vi "Mem_LvDataToMemory.vi"   [LabVIEW 2019, in "Memory Data Access.lvlib"]
uses:
  Memory Data Access.lvlib
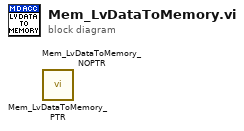
[diagram p0: block diagram]
diagram:
  n1 = call "Mem_LvDataToMemory_PTR.vi"() -> ()  [unwired: 8 in, 4 out]
  n2 = call "Mem_LvDataToMemory_NOPTR.vi"() -> ()  [unwired: 9 in, 3 out]
